vi "Fake Pelletron.vi"() -> ()   [LabVIEW 2009, in "Testing.lvlib"]
uses:
  Testing.lvlib
  interface/Pelletron.ctl
  time/Time.lvlib
  interface/Interface.lvlib
panel:
  out "error out":errorcluster
  out "Iterations":i32
  in  "stop":bool
  in  "In":T1={"Timestamp"=0, "High Voltage"=3.0, "Vacuum Pressure"=5e-07, "Column Current"=40.0, "Chain Current"=45.0, "- High Voltage Supply"=11.0, "+ High Voltage Supply"=11.5, "Radiation"=1.2, "Lost Charge"=5.0, "Control High Voltage"=3.0, "HV Control Difference"=-20.6}
  in  "Rate (Hz)":dbl=1.0
  out "Out":T1
  # "Fake Pelletron"
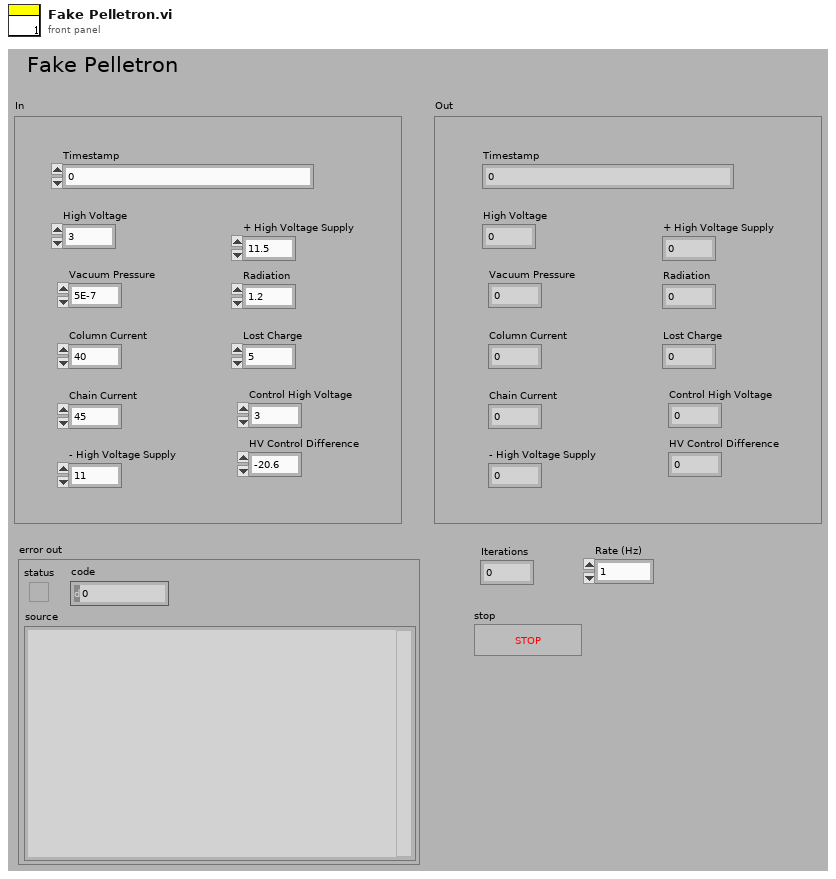
[diagram p1: front panel]
types:
  T1 = typedef "Interface.lvlib/Pelletron.ctl" = cluster{"Timestamp":u64, "High Voltage":sgl, "Vacuum Pressure":sgl, "Column Current":sgl, "Chain Current":sgl, "- High Voltage Supply":dbl, "+ High Voltage Supply":dbl, "Radiation":dbl, "Lost Charge":dbl, "Control High Voltage":dbl, "HV Control Difference":dbl}
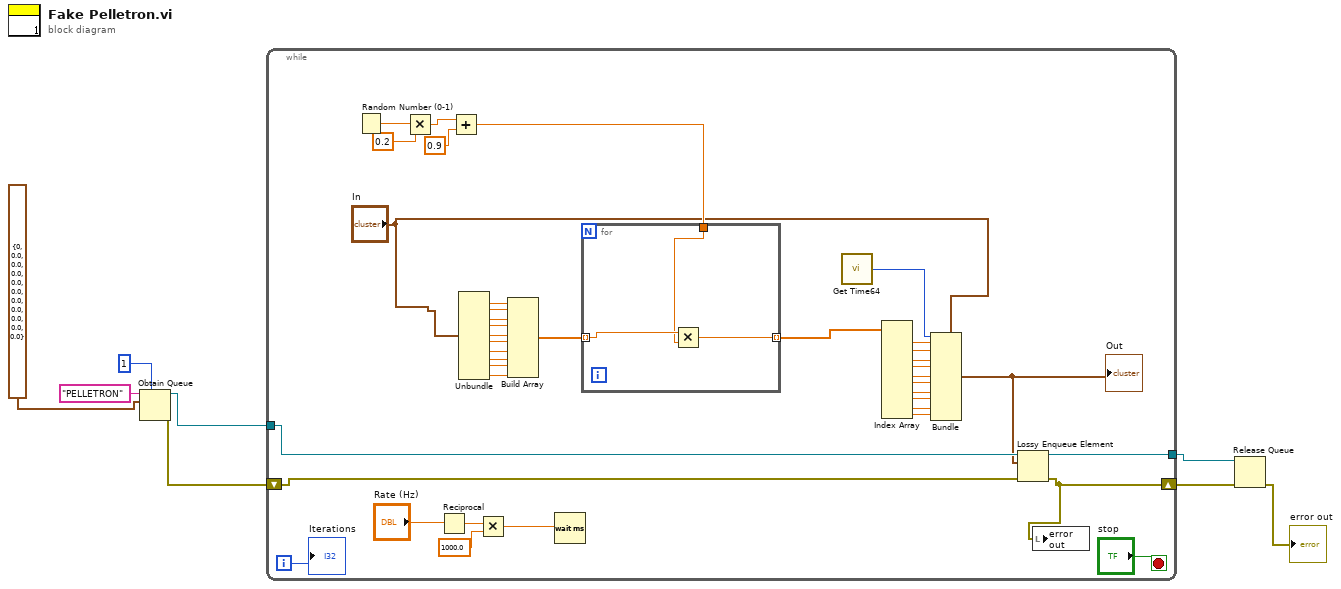
[diagram p0: block diagram]
diagram:
  n1 = Obtain Queue(max queue size (-1, unlimited)=1, name (unnamed)="PELLETRON", element data type=T1 {"Timestamp"=0, "High Voltage"=0.0, "Vacuum Pressure"=0.0, "Column Current"=0.0, "Chain Current"=0.0, "- High Voltage Supply"=0.0, "+ High Voltage Supply"=0.0, "Radiation"=0.0, "Lost Charge"=0.0, "Control High Voltage"=0.0, "HV Control Difference"=0.0} ("Cluster")) -> (queue out=w6:refnum<queue>, error out=w5:errorcluster)  [unwired: 2 in, 1 out]
  n2 = while {
    tunnel: w6 -> [w13]
    shift-right: [w9] -> w3
    shift-left: w5 -> [w12]
    tunnel: [w11] -> w2
    i -> [w14]
    stop <- "stop" stop-if-true
    n3 = Random Number (0-1)() -> (number: 0 to 1=w48:dbl)
    n4 = Multiply(x=w48, y=0.2) -> (x*y=w46:dbl)
    n5 = Reciprocal(x="Rate (Hz)") -> (1/x=w17:dbl)
    n6 = Add(x=w46, y=0.9) -> (x+y=w33:dbl)
    n7 = Unbundle("In") -> ("High Voltage"=w44:sgl, "Vacuum Pressure"=w43:sgl, "Column Current"=w42:sgl, "Chain Current"=w41:sgl, "- High Voltage Supply"=w40:dbl, "+ High Voltage Supply"=w39:dbl, "Radiation"=w38:dbl, "Lost Charge"=w37:dbl, "Control High Voltage"=w36:dbl, "HV Control Difference"=w35:dbl)  [unwired: 1 out]
    n8 = Multiply(x=w17, y=1000.0) -> (x*y=w15:dbl)
    n9 = Build Array(w44, w43, w42, w41, w40, w39, w38, w37, w36, w35) -> (w34:dbl[])
    n10 = Wait (ms)(milliseconds to wait=w15) -> ()  [unwired: 1 out]
    n11 = for {
      tunnel: w34 -> [w51] mode=indexing
      tunnel: w33 -> [w50]
      tunnel: [w49] -> w31 mode=indexing
      n12 = Multiply(x=w51, y=w50) -> (x*y=w49:dbl)
    }
    n13 = call "Get Time64.vi"() -> ("Labview time (ms)"=w19:u64)
    n14 = Index Array(array=w31) -> (element #1=w29:dbl, element #2=w28:dbl, element #3=w27:dbl, element #4=w26:dbl, element #5=w25:dbl, element #6=w24:dbl, element #7=w23:dbl, element #8=w22:dbl, element #9=w21:dbl, element #10=w20:dbl)  [unwired: 10 in]
    n15 = Bundle(cluster="In", "Timestamp"=w19, "High Voltage"=w29, "Vacuum Pressure"=w28, "Column Current"=w27, "Chain Current"=w26, "- High Voltage Supply"=w25, "+ High Voltage Supply"=w24, "Radiation"=w23, "Lost Charge"=w22, "Control High Voltage"=w21, "HV Control Difference"=w20) -> (w10:T1)
    "Out" <- w10
    n16 = Lossy Enqueue Element(queue=w13, element=w10, error in (no error)=w12) -> (queue out=w11:refnum<queue>, error out=w9:errorcluster)  [unwired: 2 out]
    n17 = local write "error out"(w9) -> ()
    "Iterations" <- w14
  }
  n18 = Release Queue(queue=w2, error in (no error)=w3) -> (error out=→"error out":errorcluster)  [unwired: 1 in, 2 out]
